vi "Add Resource Size Bytes.vi"(11 "Data in":string) -> (3 "Data out":string)   [LabVIEW 2026, in "VILab.lvlib"]
uses:
  VILab.lvlib
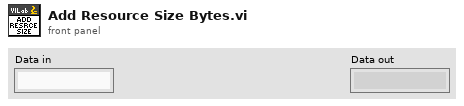
[diagram p1: front panel]
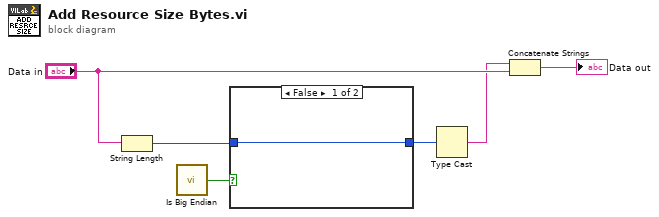
[diagram p0: block diagram]
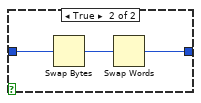
[diagram p2: hidden frame]
diagram:
  n1 = String Length(string="Data in") -> (length=w4:i32)
  n2 = call "Is Big Endian.vi"() -> ("big endian"=w6:bool)
  n3 = case shown="False" w6 {
    tunnel: [w7 w9] -> w5
    tunnel: w4 -> [w7 w8]
    frame False {
    }
    frame True {
      n4 = Swap Bytes(anything=w8) -> (byte swapped=w10:i32)
      n5 = Swap Words(1:w10) -> (0:w9:i32)
    }
  }
  n6 = Type Cast(x=w5) -> (*(type *) &x=w1:string)  [unwired: 1 in]
  n7 = Concatenate Strings(w1, "Data in") -> (→"Data out":string)
